vi "Read Stream Status.vi"(0 "device session in":refnum<class "Device Session.lvclass">, 11 "error in":errorcluster) -> (4 "device session out":refnum<class "Device Session.lvclass">, 6 "write fifo used":u32, 8 "write fifo high water":u32, 15 "error out":errorcluster)   [LabVIEW 2015, in "Device Session.lvclass"]
doc: "Reads the fullness of the sample FIFO on the FPGA.\n\n<B>Input Parameters</B>\n\n<B>device session in</B> is a reference to the session containing sessions to all instrument design libraries used in this sample project. This parameter is obtained from the 'Open Session' VI.\n\n<B>error in</B> describes error conditions that occur before this node runs. This input provides standard 'error in' functionality.\n\n<B>Output Parameters</B>\n\n<B>device session out</B> passes a reference to the session to the next VI.\n\n<B>write fifo used</B> returns the number of samples stored in the FIFO on the FPGA.\n\n<B>write fifo high water</B> returns the maximum number of samples that can be stored in the FIFO on the FPGA for the current acquisition.\n\n<B>error out</B> contains error information. This output provides standard 'error out' functionality."
uses:
  Device Session.lvclass
  Device Session.lvclass/Device Session.ctl
  FPGA Refnum.ctl
  <vilib>/Utility/error.llb/Error Cluster From Error Code.vi
  <vilib>/rvi/errors/niLvFpgaAdjustHostInterfaceError.vi
  <vilib>/rvi/interface/nirviReadWriteControl/nirviReadWriteControl.xnode
  NiFpgaLv.dll
  <vilib>/rvi/interface/Simulation/niFpgaSimulationCallBeginRW.vi
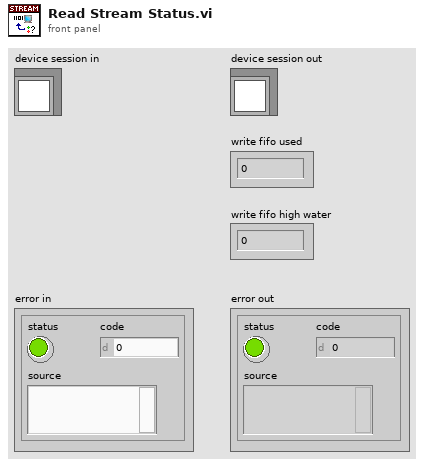
[diagram p1: front panel]
types:
  T1 = typedef "Device Session.lvclass/FPGA Refnum.ctl" = refnum<k20>
  T2 = typedef "Device Session.lvclass/Device Session Object.ctl" = cluster{"ni5171R FPGA Reference":T1, "niHSAI config":refnum<class "niHSAI Config v1 Host.lvclass">, "configured scaling coefficients":cluster{"gain":dbl, "offset":dbl}[], "number of channels to stream":u8, "selected acq channels":bool[], "number of channels":u32, "actual channel configuration":T3[], "configured channels":bool[], "sample clock rate (Hz)":dbl}
  T3 = typedef "niHSAI Types v1 Host.lvlib/Channel Configuration.ctl" = cluster{"channel":u32, "coupling":T4, "impedance":T5, "bandwidth":T6, "vertical range":dbl, "vertical offset":dbl}
  T4 = typedef "niHSAI Types v1 Host.lvlib/Coupling.ctl" = enum8{"Default", "DC", "AC"}
  T5 = typedef "niHSAI Types v1 Host.lvlib/Impedance.ctl" = enum8{"Default", "1 mega ohm", "50 ohm"}
  T6 = typedef "niHSAI Types v1 Host.lvlib/Bandwidth.ctl" = enum8{"Default", "Full Bandwidth", "Anti-alias Filter"}
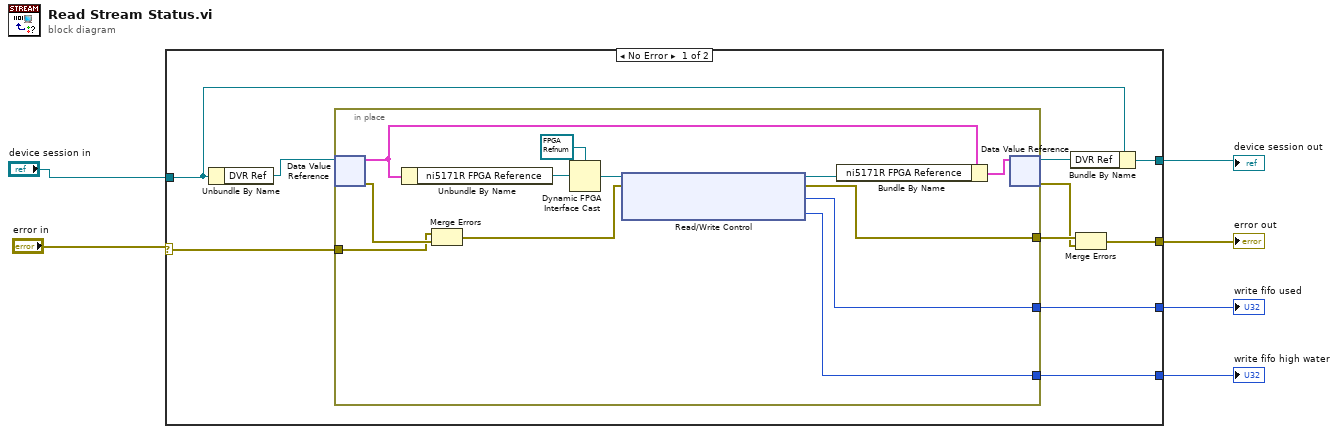
[diagram p0: block diagram]
diagram:
  n1 = case shown="No Error" "error in" {
    selector: "error in" -> [w16 w30]
    tunnel: [w11 w30] -> w3
    tunnel: "device session in" -> [w13 w29]
    tunnel: [w12 w29] -> w5
    tunnel: [w10 _] -> w2
    tunnel: [w9 _] -> w1
    frame No Error {
      n2 = Unbundle By Name(w13) -> ("DVR Ref"=w15:refnum<data-value>)
      n3 = in-place {
        in-place-border: w16 -> [w26]
        in-place-border: [w23] -> w8
        in-place-border: [w18] -> w10
        in-place-border: [w17] -> w9
        n4 = in-place-dvr #1(w15) -> (w28:T2, w27:errorcluster)
        n5 = Unbundle By Name(w28) -> ("ni5171R FPGA Reference"=w20:T1)
        n6 = Merge Errors(w26, w27) -> (w25:errorcluster)
        n7 = Dynamic FPGA Interface Cast(Session In=T1 refnum ("FPGA Interface"), Type=w20) -> (Session Out=w19:T1)
        n8 = xnode "Read/Write Control"("FPGA VI Reference In"=w19, "error in"=w25) -> ("FPGA VI Reference Out"=w24:T1, "error out"=w23:errorcluster, "status.samples in fifo"=w18:u32, "status.fifo high water (samples)"=w17:u32)
        n9 = Bundle By Name(cluster=w28, "ni5171R FPGA Reference"=w24) -> (w22:T2)
        n10 = in-place-dvr #1(w22) -> (w14:refnum<data-value>, w7:errorcluster)
      }
      n11 = Bundle By Name(cluster=w13, "DVR Ref"=w14) -> (w12:refnum<class "Device Session.lvclass">)
      n12 = Merge Errors(w8, w7) -> (w11:errorcluster)
    }
    frame Error {
    }
  }
  "error out" <- w3
  "device session out" <- w5
  "write fifo used" <- w2
  "write fifo high water" <- w1
